vi "List Sensor Names.vi"(11 "Top Level Path":path) -> (3 "Sensor Names":string[](array[string]))   [LabVIEW 2013, in "File IO.lvlib"]
uses:
  File IO.lvlib
  <vilib>/xml/Load XML File.vi
  <vilib>/xml/Close Reference(Node).vi
  <vilib>/xml/NI_XML.lvlib
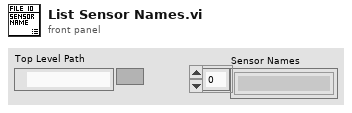
[diagram p1: front panel]
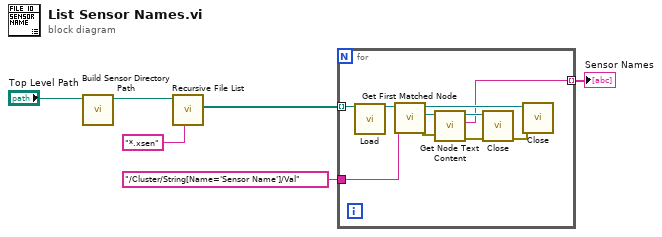
[diagram p0: block diagram]
diagram:
  n1 = call "Build Sensor Directory Path.vi"("Top Level Path"="Top Level Path") -> ("Sensor Directory Path"=w3:path)  [unwired: 10 in]
  n2 = call <vilib>:"Recursive File List.vi"("pattern"="*.xsen", "Folder Path"=w3) -> ("All Files in Dir"=w5:path[])  [unwired: 5 in, 4 out]
  n3 = for {
    tunnel: w5 -> [w14] mode=indexing
    tunnel: "/Cluster/String[Name='Sensor Name']/Val" -> [w15]
    tunnel: [w8] -> w1 mode=indexing
    n4 = call-poly <vilib>:"Load.vi"("path to XML document"=w14) -> ("DOM document out"=w16:refnum<k20>)  [unwired: 12 in, 2 out]
    n5 = call <vilib>:"Get First Matched Node.vi"("XPath expression"=w15, "node in"=w16) -> ("error out"=w9:errorcluster, "node result"=w12:refnum<k20>, "node out"=w13:refnum<k20>)  [unwired: 7 in]
    n6 = call <vilib>:"Get Node Text Content.vi"("error in (no error)"=w9, "node in"=w12) -> ("error out"=w10:errorcluster, "node text"=w8:string, "node out"=w11:refnum<k20>)  [unwired: 7 in]
    n7 = call-poly <vilib>:"Close.vi"("error in (no error)"=w10, "node"=w11) -> ("error out"=w7:errorcluster)  [unwired: 7 in]
    n8 = call-poly <vilib>:"Close.vi"("error in (no error)"=w7, "node"=w13) -> ()  [unwired: 7 in, 1 out]
  }
  "Sensor Names" <- w1
